vi "NIVS Print Debug String.vi"(6 "Color (Plain White)":u16(ring)=7 items=["Plain White"=7, "Bold White"=15, "Bold Blue"=9, "Bold Green"=10, "Bold Red"=12], 7 "error in (no error)":errorcluster, 8 "Add to NIVS Log FIle? (T)":bool=TRUE, 9 "Append EOL? (T)":bool=TRUE, 10 "Debug String":string) -> (0 "error out":errorcluster)   [LabVIEW 2019, in "GE_RM_Real Time.lvlib"]
doc: "Prints a string to the console and optionally to NI VeriStand's data log.\n\nThis VI functions in Windows and RT and does not depend on ni_emb.dll. This VI only works when run within the context of NI VeriStand's engine."
uses:
  GE_RM_Real Time.lvlib
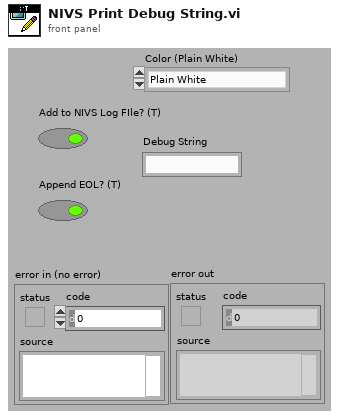
[diagram p1: front panel]
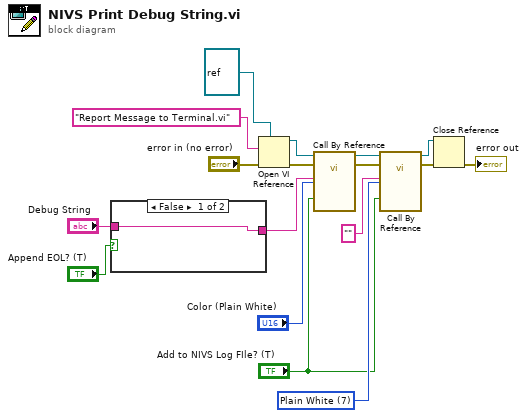
[diagram p0: block diagram]
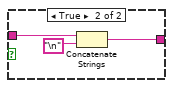
[diagram p2: hidden frame]
diagram:
  w13 = u16 7 items=["Plain White"=7, "Bold White"=15, "Bold Blue"=9, "Bold Green"=10, "Bold Red"=12] ("Color (Plain White)")
  n1 = case shown="False" "Append EOL? (T)" {
    tunnel: [w18 w21] -> w12
    tunnel: "Debug String" -> [w18 w20]
    frame False {
    }
    frame True {
      n2 = Concatenate Strings(w20, "\n") -> (w21:string)
    }
  }
  n3 = Open VI Reference(type specifier VI Refnum (for type only)=refnum<vi> refnum, vi path="Report Message to Terminal.vi", error in (no error)="error in (no error)") -> (vi reference=w11:refnum<vi>, error out=w10:errorcluster)  [unwired: 3 out]
  n4 = call-by-ref "?"(reference=w11, error in=w10, "Add to log file? (T)"="Add to NIVS Log FIle? (T)", "Color (Plain White)"="Color (Plain White)", "Message"=w12) -> (reference out=w8:refnum<vi>, error out=w7:errorcluster)  [unwired: 8 in, 1 out]
  n5 = call-by-ref "?"(reference=w8, error in=w7, "Add to log file? (T)"="Add to NIVS Log FIle? (T)", "Color (Plain White)"=w13, "Message"="") -> (reference out=w14:refnum<vi>, error out=w15:errorcluster)  [unwired: 8 in, 1 out]
  n6 = Close Reference(reference=w14, error in (no error)=w15) -> (error out=→"error out":errorcluster)
